vi "tempallgetPID.vi"(1 "Neocera: Heater or Analog;\nLakeshore: Heater 1 or 2":u16(ring)=1 items=["Heater / Heater 1"=1, "Analog / Heater 2"=2], 2 "Temperature controller":u16(ring) items=["Lakeshore 336", "Conductus/Neocera"], 3 "GPIB address":string="11") -> (0 "Out":string="P=499.99;I=2.;D=0.0;")   [LabVIEW 2014]
panel:
  out "error out":errorcluster
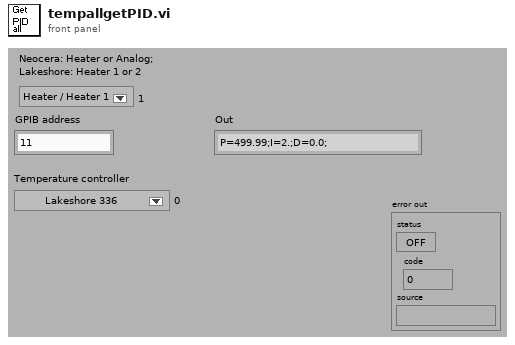
[diagram p1: front panel]
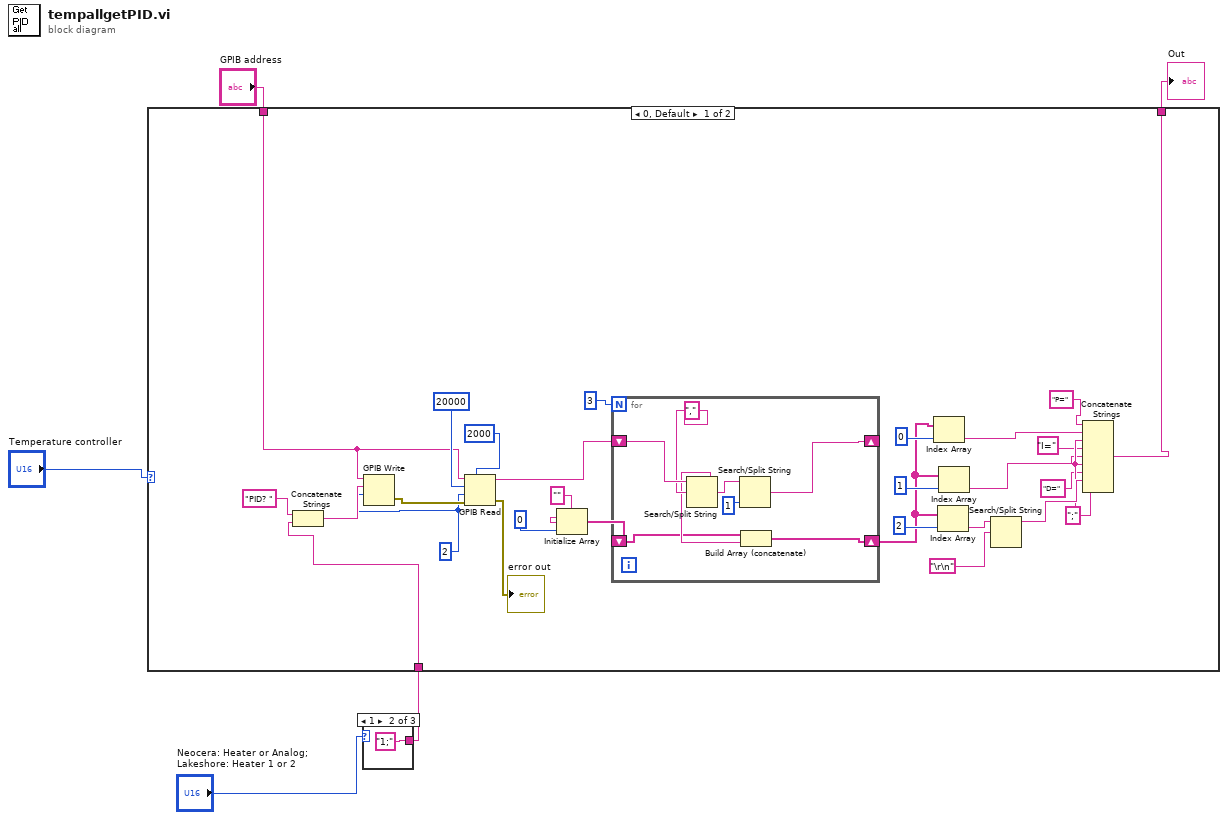
[diagram p0: block diagram]
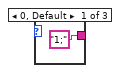
[diagram p2: hidden frame]
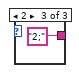
[diagram p3: hidden frame]
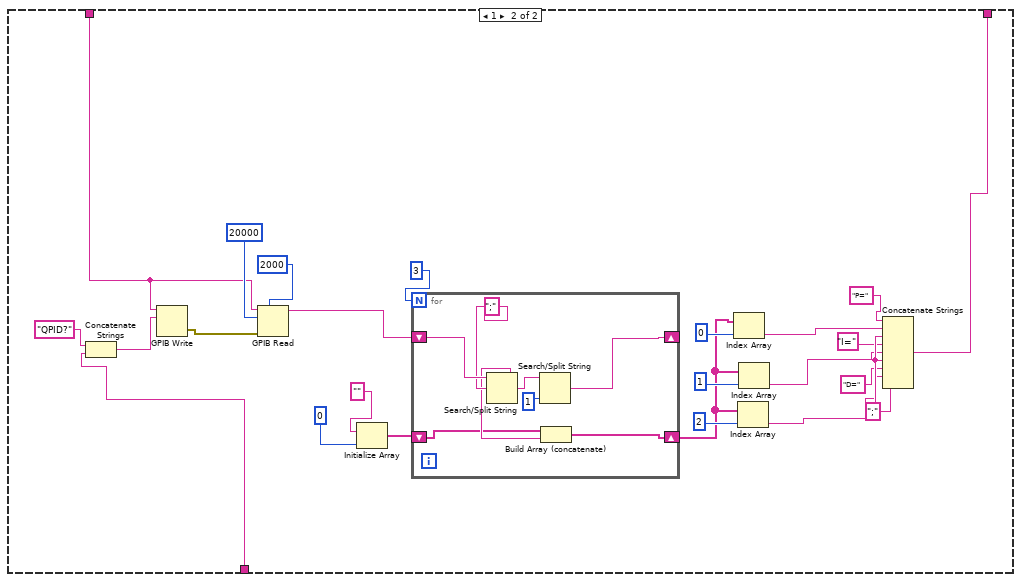
[diagram p4: hidden frame]
diagram:
  n1 = case shown="1" "Neocera: Heater or Analog;\nLakeshore: Heater 1 or 2" {
    tunnel: ["1;" "1;" "2;"] -> w4
    frame 0, Default {
    }
    frame 1 {
    }
    frame 2 {
    }
  }
  n2 = case shown="0, Default" "Temperature controller" {
    tunnel: w4 -> [w13 w46]
    tunnel: "GPIB address" -> [w12 w47]
    tunnel: [w11 w45] -> w2
    frame 0, Default {
      w10 = 2
      w33 = ";"
      n3 = Concatenate Strings("PID? ", w13) -> (w16:string)
      n4 = GPIB Write(0:w12, 1:w16, 2:w10) -> (6:w14:errorcluster)  [unwired: 2 in, 1 out]
      n5 = GPIB Read(0:w12, 1:20000, 2:w10, 3:w14, 4:2000) -> (5:w20:string, 7:→"error out":errorcluster)  [unwired: 1 out]
      n6 = Initialize Array("", 0) -> (w21:string[])
      n7 = for {
        N: 3 -> [_]
        shift-right: [w41] -> _
        shift-left: w20 -> [w44]
        shift-right: [w37] -> w24
        shift-left: w21 -> [w38]
        n8 = Search/Split String(string=w44, search string/char (-)=",") -> (substring before match=w39:string, match + rest of string=w40:string)  [unwired: 1 in, 1 out]
        n9 = Search/Split String(string=w40, offset (0)=1) -> (match + rest of string=w41:string)  [unwired: 1 in, 2 out]
        n10 = Build Array (concatenate)(w38, w39) -> (w37:string[])
      }
      n11 = Index Array(array=w24, index=0) -> (element=w29:string)
      n12 = Index Array(array=w24, index=2) -> (element=w34:string)
      n13 = Index Array(array=w24, index=1) -> (element=w31:string)
      n14 = Search/Split String(string=w34, search string/char (-)="\r\n") -> (substring before match=w36:string)  [unwired: 1 in, 2 out]
      n15 = Concatenate Strings("P=", w29, w33, "I=", w31, w33, "D=", w36, w33) -> (w11:string)
    }
    frame 1 {
      w68 = ";"
      n16 = Concatenate Strings("QPID?", w46) -> (w50:string)
      n17 = GPIB Write(0:w47, 1:w50) -> (6:w48:errorcluster)  [unwired: 3 in, 1 out]
      n18 = GPIB Read(0:w47, 1:20000, 3:w48, 4:2000) -> (5:w54:string)  [unwired: 1 in, 2 out]
      n19 = Initialize Array("", 0) -> (w55:string[])
      n20 = for {
        N: 3 -> [_]
        shift-right: [w73] -> _
        shift-left: w54 -> [w76]
        shift-right: [w69] -> w58
        shift-left: w55 -> [w70]
        n21 = Search/Split String(string=w76, search string/char (-)=";") -> (substring before match=w71:string, match + rest of string=w72:string)  [unwired: 1 in, 1 out]
        n22 = Search/Split String(string=w72, offset (0)=1) -> (match + rest of string=w73:string)  [unwired: 1 in, 2 out]
        n23 = Build Array (concatenate)(w70, w71) -> (w69:string[])
      }
      n24 = Index Array(array=w58, index=0) -> (element=w63:string)
      n25 = Index Array(array=w58, index=2) -> (element=w67:string)
      n26 = Index Array(array=w58, index=1) -> (element=w65:string)
      n27 = Concatenate Strings("P=", w63, w68, "I=", w65, w68, "D=", w67, w68) -> (w45:string)
    }
  }
  "Out" <- w2
